vi "Main.vi"(8 "Error In":errorcluster, 9 "Pop-up New Error Dialogue Setting (Default = Pop-up Dialogue)":T1, 10 "The folder to store the Error Logs":path, 11 "Test Rig Name or Acronym":string) -> (0 "Error Out":errorcluster)   [LabVIEW 2023, in "Error Manager.lvlib"]
doc: "Error Manager. Asynchronous Module. User-facing GUI. Logs all errors to a log file.\n\nRecommended use: \n1. Start the Error Manager by calling this VI at application start prior to other asynchronous modules being started and prior to other start-up actions being performed (for example, prior to retrieving settings or limits from a file or from a database). This ensures that all parts of the app can report to the Error Manager any errors encountered during app start-up.\n\n2. Use Public API VIs to interact with this VI. For example, call 'Handle Error' to report an error to the asynchronous Error Manager module, or call 'Show Front Panel' to pop-up the Error Manager GUI to the user.\n\n3. Close the Error Manager by calling 'Close Module' during app shutdown, after all other shutdown operations have been completed (for example, after all other asynchronous modules have been stopped). This enables the Error Manager to log any errors that may happen during app shutdown.\n\nError in behaviour: This VI skips execution (does not execute) if 'error in' contains an error."
uses:
  Error Manager.lvlib
  Pop-up New Error Dialogue Setting (enum).ctl
  MHL Queue/Command (enum).ctl
  LogToFileQueue/Command (enum).ctl
  NewErrorDialogueLoopQueue/Command (enum).ctl
  New Error Dialogue GUI/New Error (To Be Displayed To User) (cluster).ctl
  Error Log/Error to be logged (cluster).ctl
  Error Log/Error Type (enum).ctl
  Reported Error (cluster).ctl
  Pop-up New Error Dialogue Instruction (enum).ctl
  Read-Unread Status (enum).ctl
  Error in current one-second interval (cluster).ctl
  <vilib>/Utility/error.llb/DialogType.ctl
  Error Log/ErrorLog.lvlib
  MHL Queue/MHL Queue.lvlib
  LogToFileQueue/LogToFileQueue.lvlib
  NewErrorDialogueLoopQueue/NewErrorDialogueLoopQueue.lvlib
  New Error Dialogue GUI/New Error Dialogue GUI.lvlib
panel:
  in  "Sizing Tool":bool
  in  "Mark error as read":bool
  in  "Mark all errors as read":bool
  in  "Display Order ComboBox":string(combo) caption="Display Order"
  out "Error Out":errorcluster
  in  "Open Error Logs Folder":bool
  in  "Open Error Log in Notepad":bool
  out "Error Log Filepath":string
  out "Full Error Message":string caption="Error Message Of Selected Error"
  in  "MCL":i32[](listbox) caption="Errors since app started"
  out "Close module?":bool
  out "EHL iteration":i32
  out "MHL iteration":i32
  out "Error Out":errorcluster
  # "The region below is invisible to the user. For developer use only."
  # "Input\nInputs to the VI"
  # "Development\ncontrols/indicators useful for development and testing, but which are not outputs of the VI"
  # "Output\nOutputs of the VI"
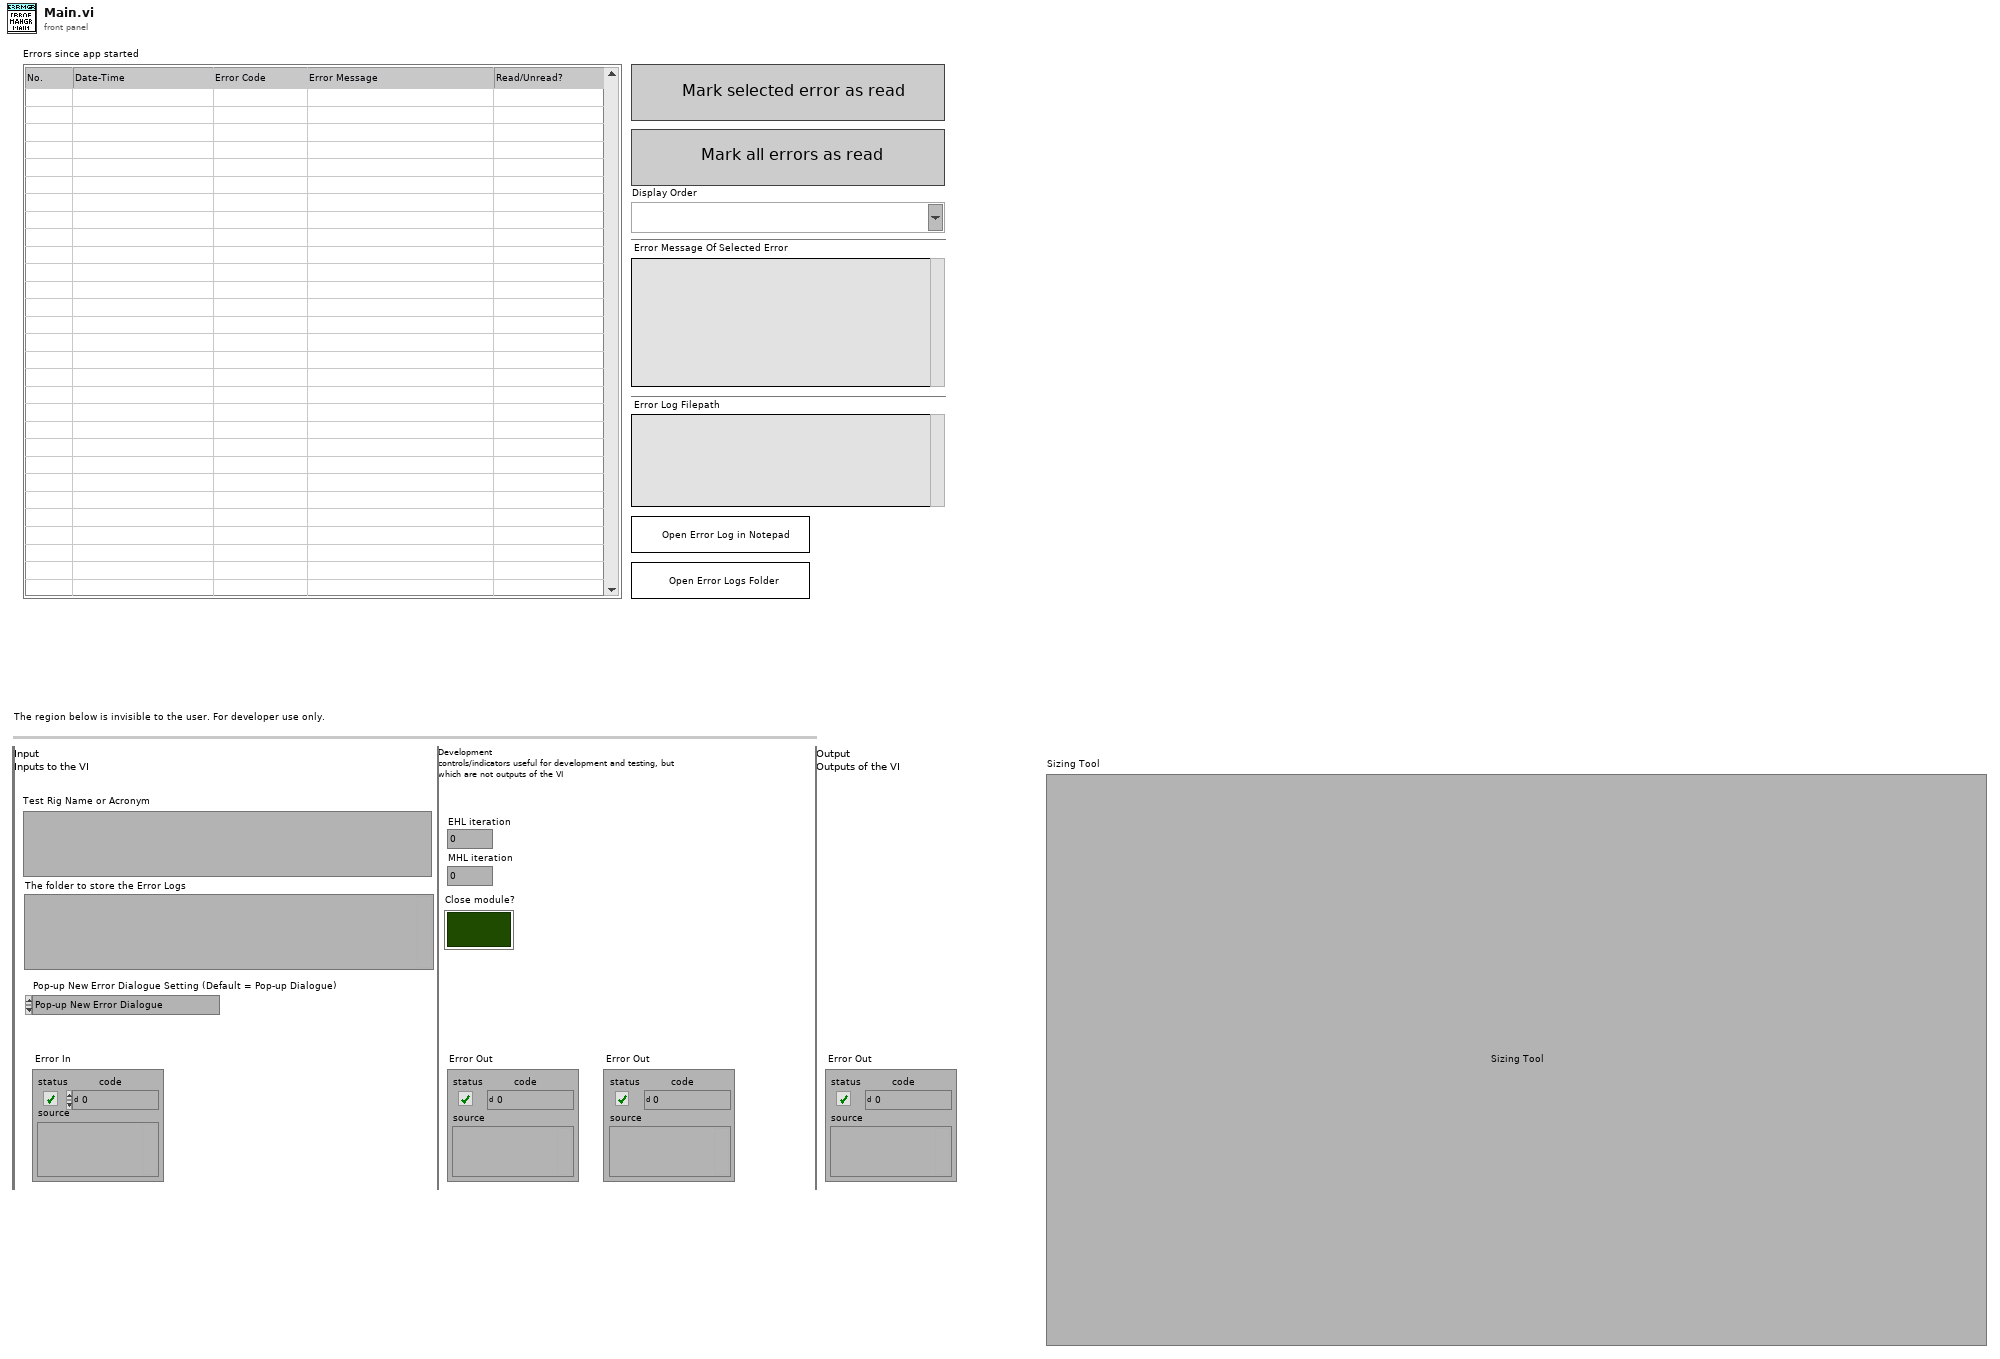
[diagram p1: front panel]
types:
  T1 = typedef "Error Manager.lvlib/Pop-up New Error Dialogue Setting (enum).ctl" = enum16{"Pop-up New Error Dialogue", "Don't pop-up New Error Dialogue"}
  T2 = typedef "Error Manager.lvlib/NewErrorDialogueLoopQueue.lvlib/Command (enum).ctl" = enum16{"Init Loop", "Close Loop", "Pop-up New Error Dialogue"}
  T3 = typedef "Error Manager.lvlib/LogToFileQueue.lvlib/Command (enum).ctl" = enum16{"Init Loop", "Close Loop", "Log Error"}
  T4 = typedef "Error Manager.lvlib/MHL Queue.lvlib/Command (enum).ctl" = enum16{"Init Module", "Close Module", "Internal Error", "Create Error Log File", "Show Front Panel", "Handle Error", "Refresh MCL", "MCL Value Change", "Mark Error As Read", "Mark All Errors As Read", "Change Display Order", "One-Second Interval Expired"}
  T5 = typedef "Error Manager.lvlib/ErrorLog.lvlib/Error to be logged (cluster).ctl" = cluster{"Error Type":T6, "Error Number":i32, "Timestamp":timestamp, "Error code":i32, "Error message":string}
  T6 = typedef "Error Manager.lvlib/ErrorLog.lvlib/Error Type (enum).ctl" = enum16{"New", "Identical to last logged error"}
  T7 = typedef "Error Manager.lvlib/Reported Error (cluster).ctl" = cluster{"Timestamp":timestamp, "Error code":i32, "Error message":string, "Pop-up New Error Dialogue Instruction":T8}
  T8 = typedef "Error Manager.lvlib/Pop-up New Error Dialogue Instruction (enum).ctl" = enum16{"Let Error Manager Decide (Default)", "Don't pop-up", "Pop-up"}
  T9 = typedef "Error Manager.lvlib/Read-Unread Status (enum).ctl" = enum16{"Unread", "Read"}
  T10 = typedef "Error Manager.lvlib/Module Data (cluster).ctl" = cluster{"Total no. of errors reported":i32, "Total no. of errors handled":i32, "Latest Handled Errors (chronological order)":T11[], "Display Order":T12, "Errors in current one-second interval":T13[], "ErrorMarkedAsRead":bool[]}
  T11 = typedef "Error Manager.lvlib/Handled Error (cluster).ctl" = cluster{"Error Number":i32, "Timestamp":timestamp, "Error code":i32, "Error message":string, "Read-Unread Status":T9}
  T12 = typedef "Error Manager.lvlib/Display Order (enum).ctl" = enum16{"Most Recent First (inverse-chronological)", "Oldest First (chronological)"}
  T13 = typedef "Error Manager.lvlib/Error in current one-second interval (cluster).ctl" = cluster{"Error code":i32, "No. of times error reported":u32, "No. of times error handled":u32}
  T14 = typedef "Error Manager.lvlib/New Error Dialogue GUI.lvlib/New Error (To Be Displayed To User) (cluster).ctl" = cluster{"Error Code":i32, "Error Message":string}
  T15 = typedef "DialogType.ctl" = u16
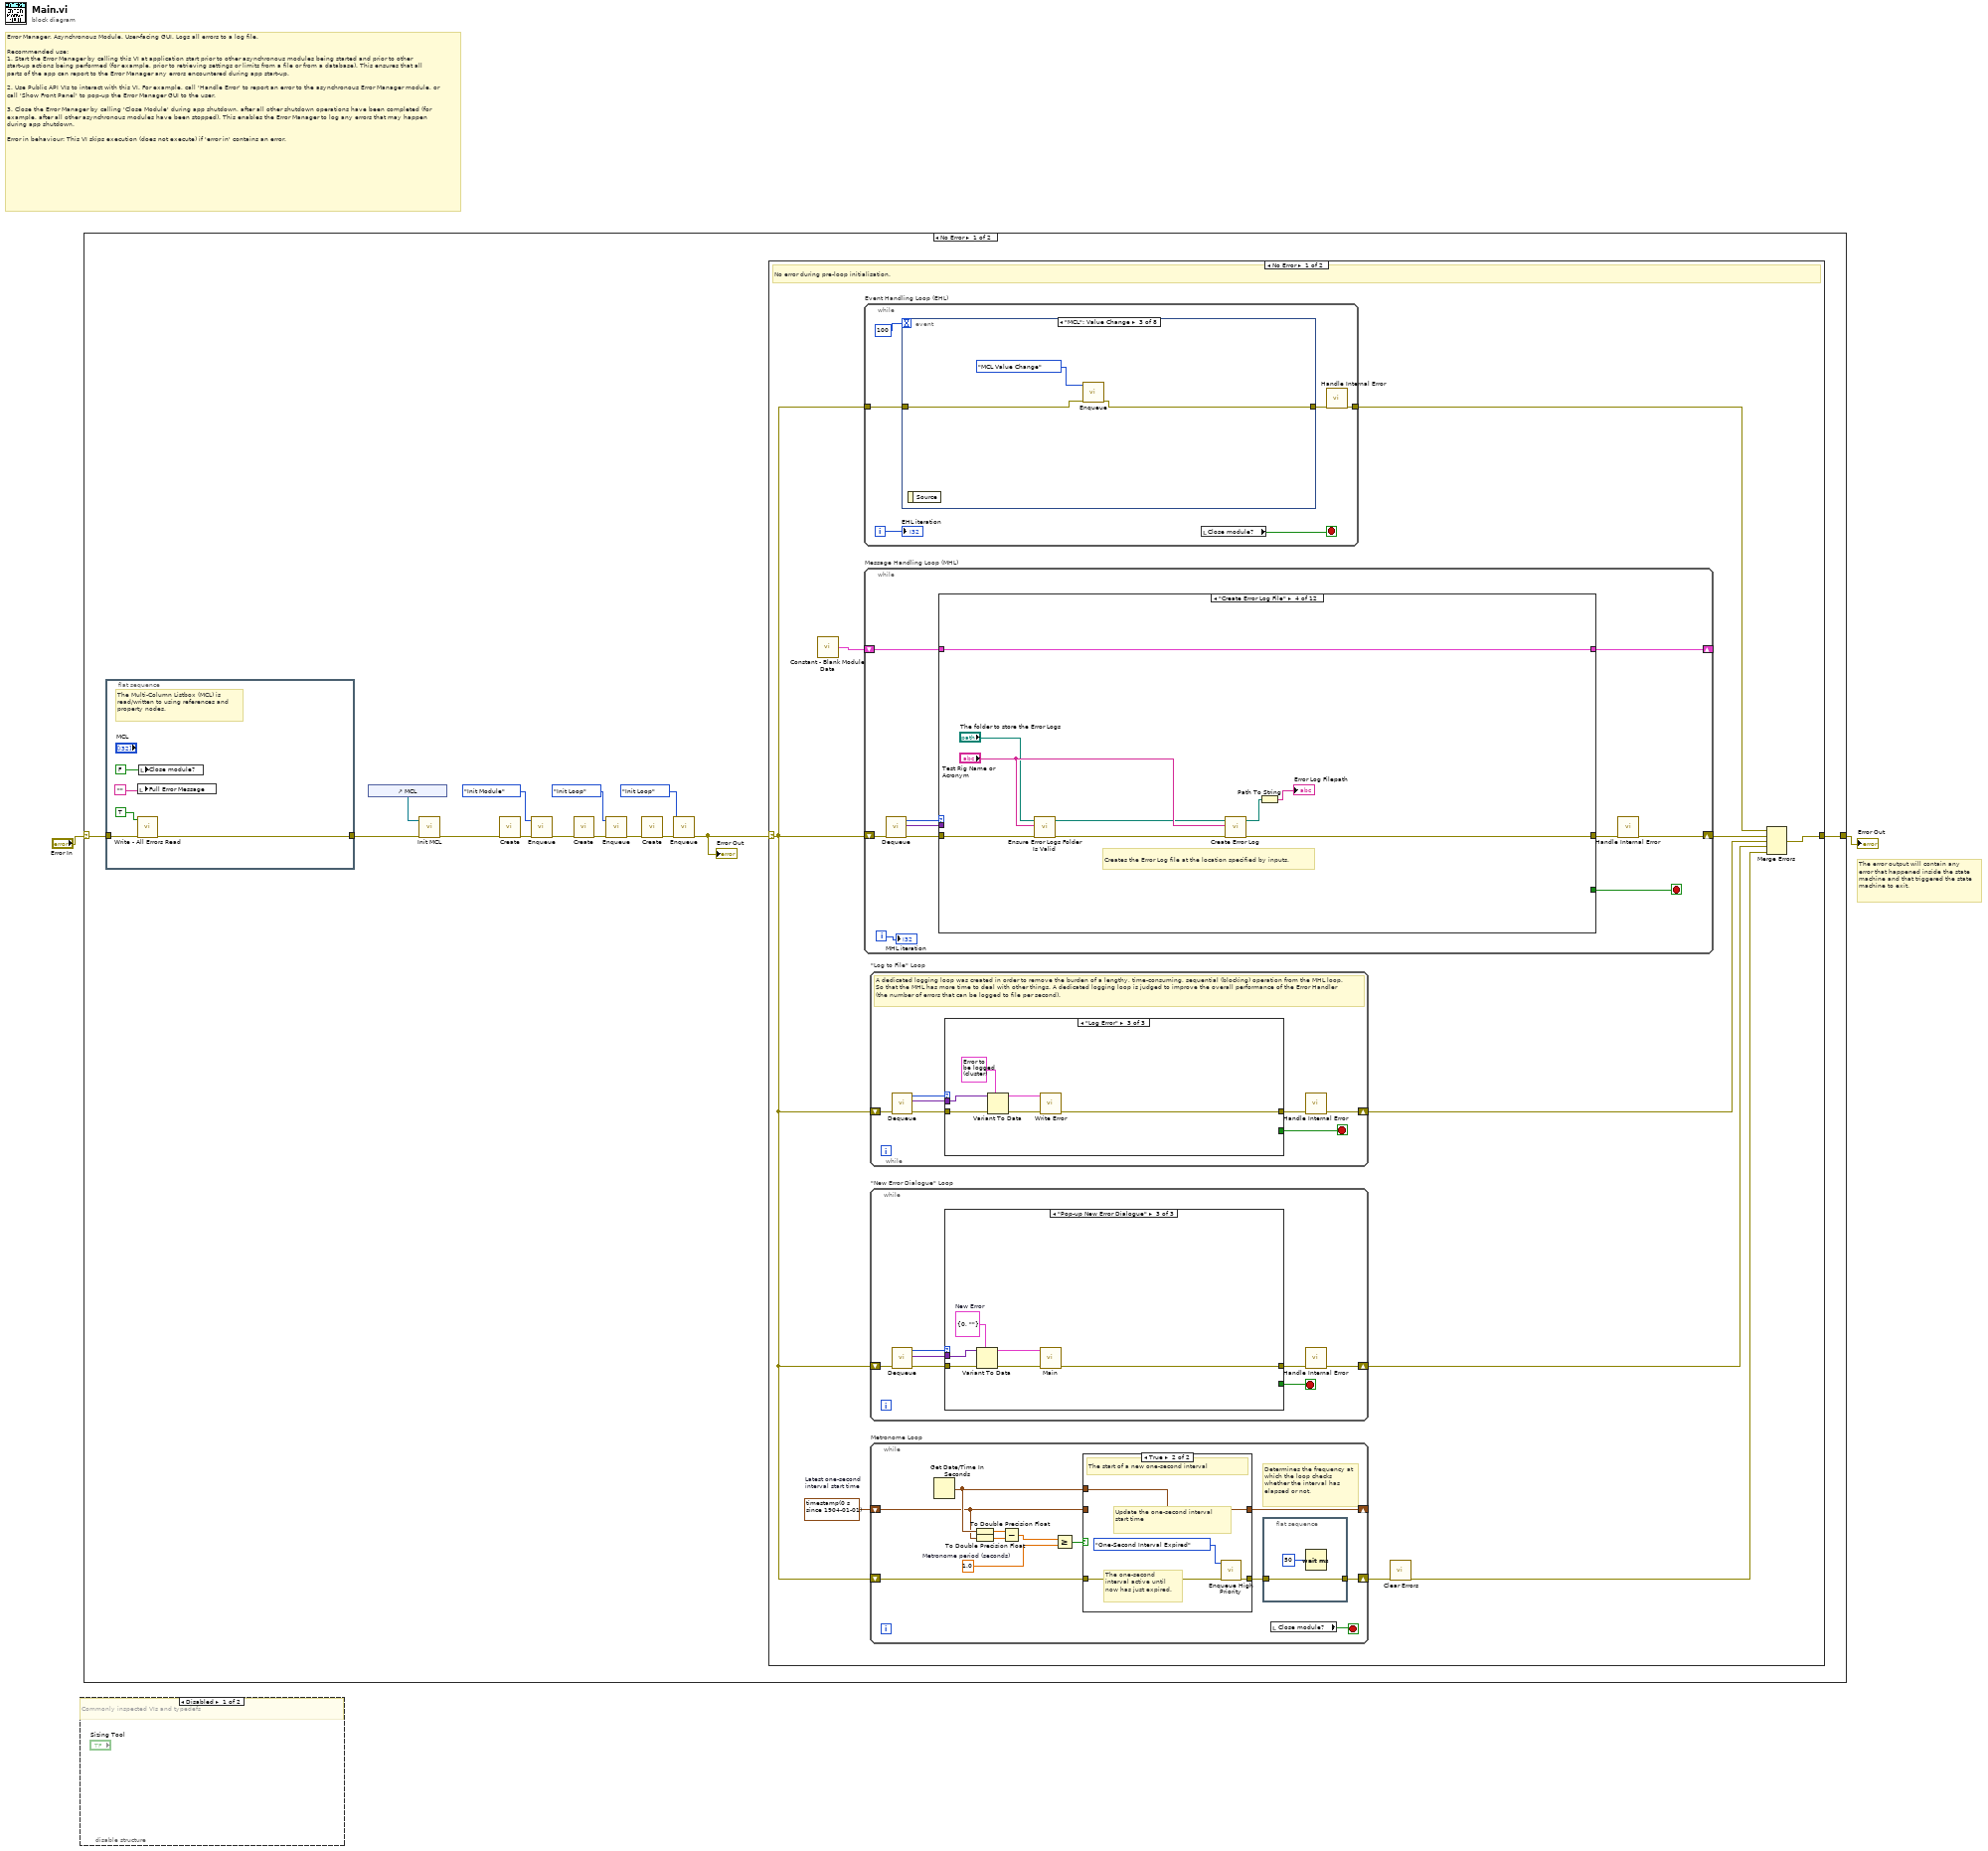
[diagram p0: block diagram]
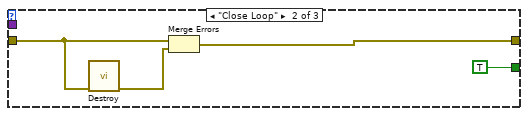
[diagram p3: hidden frame]
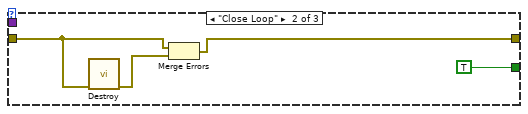
[diagram p5: hidden frame]
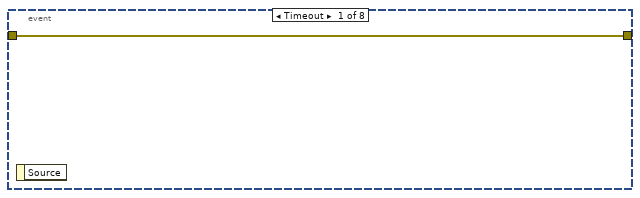
[diagram p6: hidden frame]
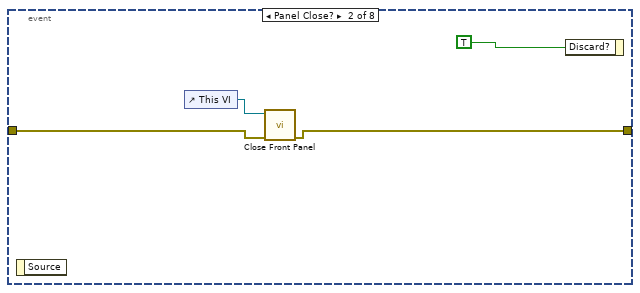
[diagram p7: hidden frame]
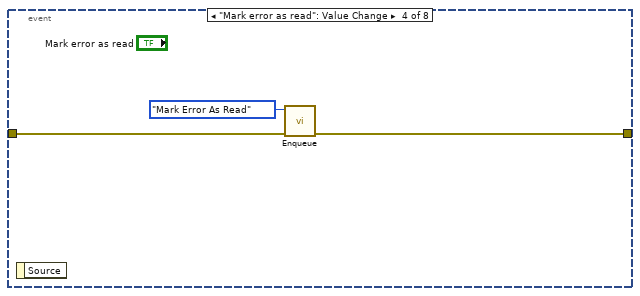
[diagram p8: hidden frame]
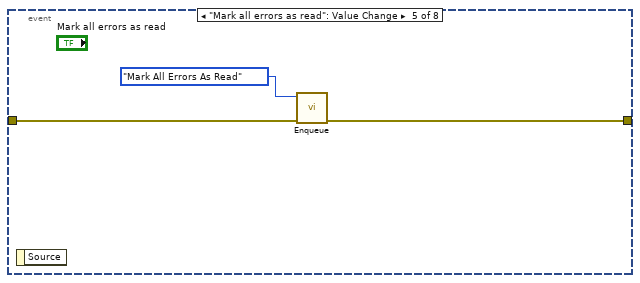
[diagram p9: hidden frame]
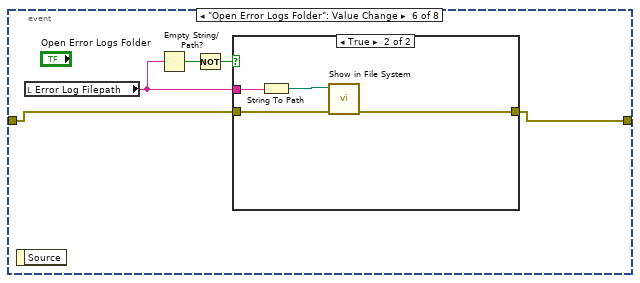
[diagram p10: hidden frame]
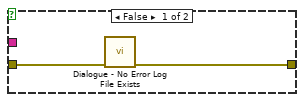
[diagram p11: hidden frame]
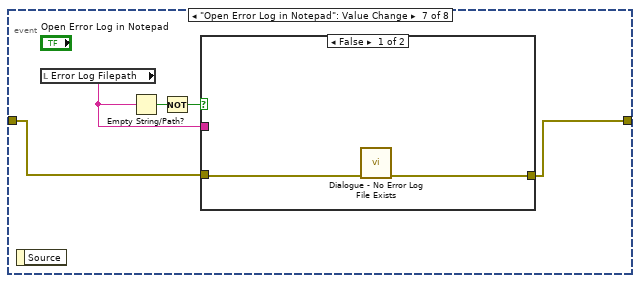
[diagram p12: hidden frame]
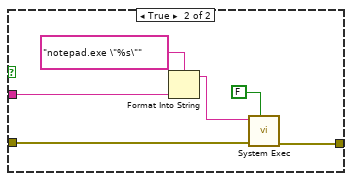
[diagram p13: hidden frame]
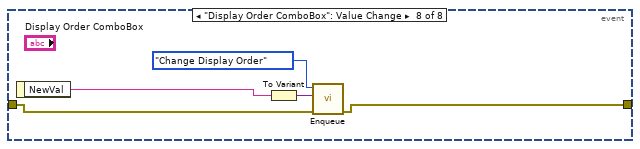
[diagram p14: hidden frame]
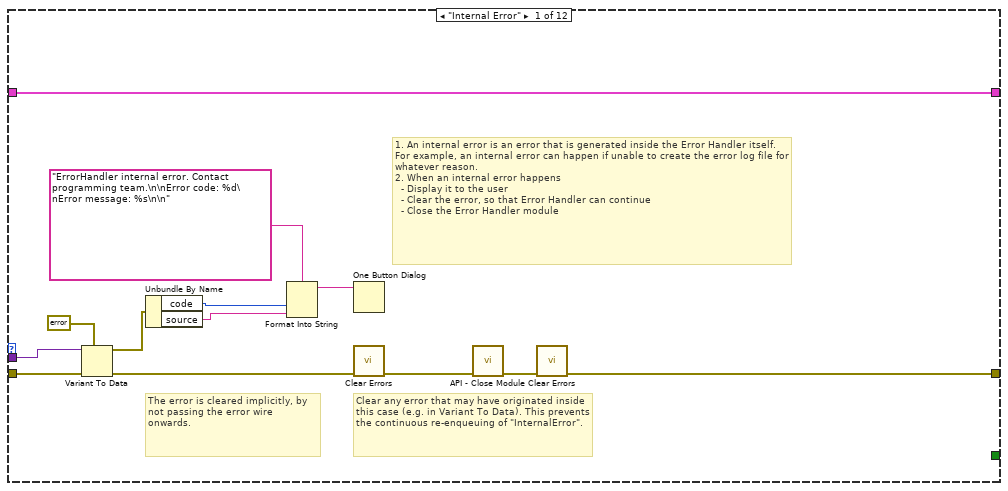
[diagram p15: hidden frame]
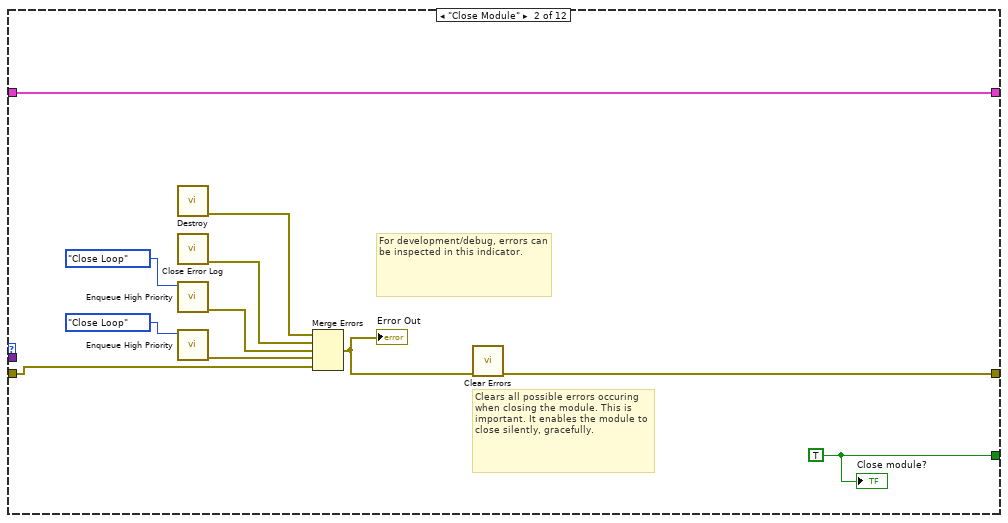
[diagram p16: hidden frame]
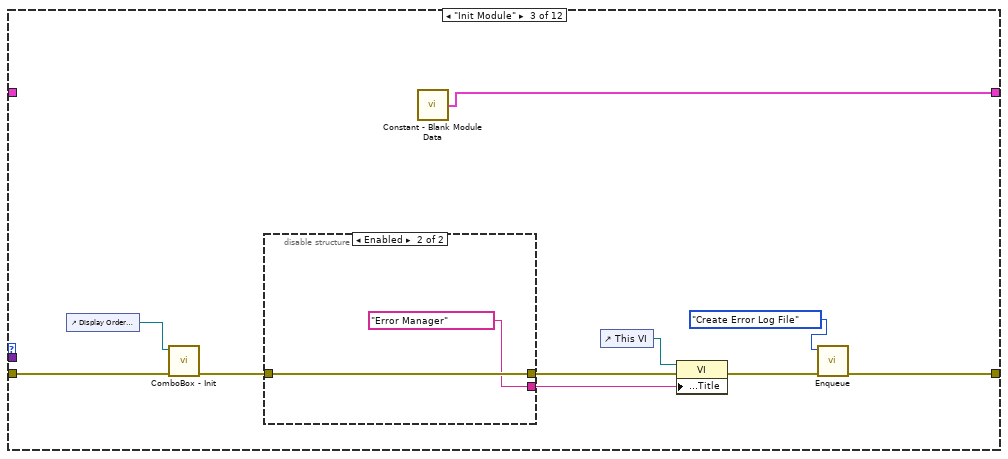
[diagram p17: hidden frame]
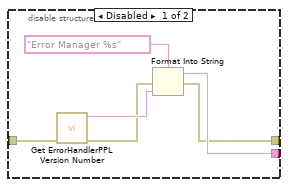
[diagram p18: hidden frame]
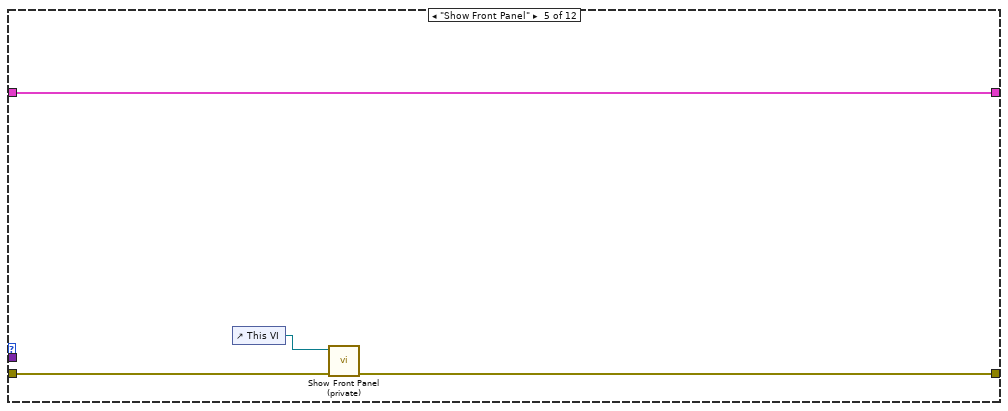
[diagram p19: hidden frame]
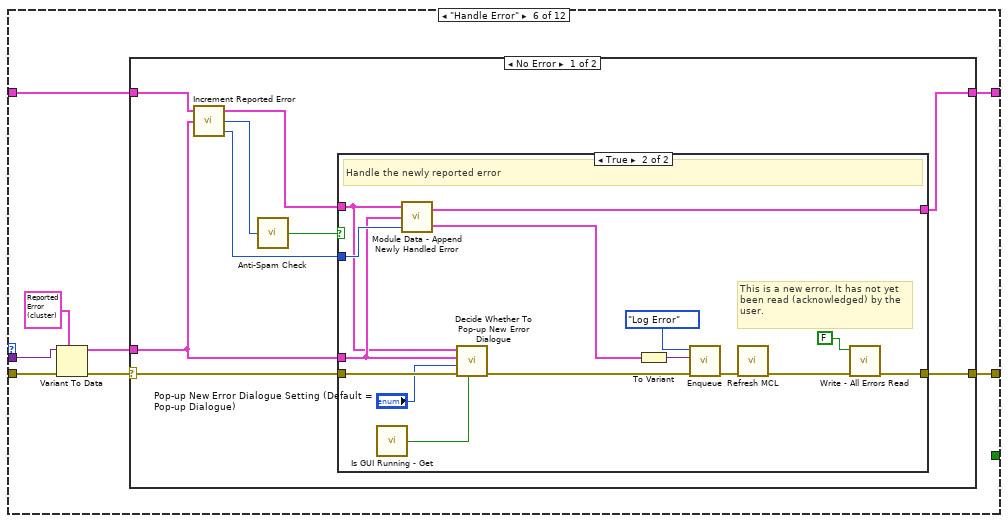
[diagram p20: hidden frame]
diagram:
  # "The error output will contain any error that happened inside the state machine and that triggered the state machine to exit."
  # "Error Manager. Asynchronous Module. User-facing GUI. Logs all errors to a log file.\n\nRecommended use: \n1. Start the Error Manager by calling this VI at application start prior to other asynchronous modules being started and prior to other start-up actions being performed (for example, prior to retrieving settings or limits from a file or from a database). This ensures that all parts of the app can report to the Error Manager any errors encountered during app start-up.\n\n2. Use Public API VIs to interact with this VI. For example, call 'Handle Error' to report an error to the asynchronous Error Manager module, or call 'Show Front Panel' to pop-up the Error Manager GUI to the user.\n\n3. Close the Error Manager by calling 'Close Module' during app shutdown, after all other shutdown operations have been completed (for example, after all other asynchronous modules have been stopped). This enables the Error Manager to log any errors that may happen during app shutdown.\n\nError in behaviour: This VI skips execution (does not execute) if 'error in' contains an error."
  n1 = disable-structure shown="Disabled" {
    frame Disabled {
      # "Commonly inspected VIs and typedefs"
    }
    frame Enabled {
    }
  }
  n2 = case shown="No Error" "Error In" {
    selector: "Error In" -> [w13 w377]
    tunnel: [w16 w377] -> w2
    frame No Error {
      n3 = flat-sequence {
        tunnel: [w20] -> w11
        tunnel: w13 -> [w19]
        frame #0 {
          # "The Multi-Column Listbox (MCL) is read/written to using references and property nodes."
          n4 = call "Write - All Errors Read.vi"("error in (no error)"=w19, "All Errors Read?"=TRUE) -> ("error out"=w20:errorcluster)  [unwired: 9 in]
          n5 = local write "Full Error Message"("") -> ()
          n6 = local write "Close module?"(FALSE ("Close module?")) -> ()
        }
      }
      n7 = control-ref of="MCL"() -> (w12:refnum<vi>)
      n8 = call "Init MCL.vi"("error in (no error)"=w11, "MCL Reference"=w12) -> ("error out"=w10:errorcluster)  [unwired: 9 in]
      n9 = call "Create.vi"("error in (no error)"=w10) -> ("error out"=w15:errorcluster)  [unwired: 10 in]
      n10 = call "Enqueue.vi"("error in (no error)"=w15, "Command"=Command_(enum)."Init Module") -> ("error out"=w14:errorcluster)  [unwired: 9 in]
      n11 = call "Create.vi"("error in (no error)"=w14) -> ("error out"=w8:errorcluster)  [unwired: 10 in]
      n12 = call "Enqueue.vi"("error in (no error)"=w8, "Command"=Command_(enum)."Init Loop") -> ("error out"=w7:errorcluster)  [unwired: 9 in]
      n13 = call "Create.vi"("error in (no error)"=w7) -> ("error out"=w5:errorcluster)  [unwired: 10 in]
      n14 = call "Enqueue.vi"("error in (no error)"=w5, "Command"=Command_(enum)."Init Loop") -> ("error out"=w4:errorcluster)  [unwired: 9 in]
      "Error Out" <- w4
      n15 = case shown="No Error" w4 {
        selector: w4 -> [w24 w376]
        tunnel: [w30 w375] -> w16
        frame No Error {
          w28 = timestamp(0 s since 1904-01-01)  # Latest one-second interval start time
          # "No error during pre-loop initialisation."
          n16 = call "Constant - Blank Module Data.vi"() -> ("Blank Module Data"=w26:T10)
          n17 = while "Event Handling Loop (EHL)" {
            tunnel: w24 -> [w70]
            tunnel: [w68] -> w29
            i -> [w73]
            stop <- w71 stop-if-true
            n18 = event shown="[2] \"MCL\": Value Change" {
              selector: _ -> [_ _ _ _ _ _ _ _]
              dyn-events: _ -> [_ _ _ _ _ _ _ _]
              timeout: 100 -> [_ _ _ _ _ _ _ _]
              tunnel: w70 -> [w74 w76 w81 w84 w87 w89 w100 w116]
              tunnel: [w74 w75 w80 w83 w86 w88 w99 w115] -> w69
              event Timeout {
                n19 = event-data() -> ()  [unwired: 1 in, 1 out]
              }
              event Panel Close? {
                n20 = event-data() -> ()  [unwired: 1 in, 1 out]
                n21 = control-ref of="This VI"() -> (w77:refnum<vi>)
                n22 = call "Close Front Panel.vi"("Error In"=w76, "VI Reference"=w77) -> ("Error Out"=w75:errorcluster)  [unwired: 9 in]
                n23 = event-data("Discard?"=TRUE) -> ()  [unwired: 1 in, 1 out]
              }
              event "MCL": Value Change {
                n24 = event-data() -> ()  [unwired: 1 in, 1 out]
                n25 = call "Enqueue.vi"("error in (no error)"=w81, "Command"=Command_(enum)."MCL Value Change") -> ("error out"=w80:errorcluster)  [unwired: 9 in]
              }
              event "Mark error as read": Value Change {
                n26 = event-data() -> ()  [unwired: 1 in, 1 out]
                n27 = call "Enqueue.vi"("error in (no error)"=w84, "Command"=Command_(enum)."Mark Error As Read") -> ("error out"=w83:errorcluster)  [unwired: 9 in]
              }
              event "Mark all errors as read": Value Change {
                n28 = event-data() -> ()  [unwired: 1 in, 1 out]
                n29 = call "Enqueue.vi"("error in (no error)"=w87, "Command"=Command_(enum)."Mark All Errors As Read") -> ("error out"=w86:errorcluster)  [unwired: 9 in]
              }
              event "Open Error Logs Folder": Value Change {
                n30 = event-data() -> ()  [unwired: 1 in, 1 out]
                n31 = local read "Error Log Filepath"() -> (w90:string)
                n32 = Empty String/Path?(string/path=w90) -> (empty?=w92:bool)
                n33 = Not(x=w92) -> (.not. x?=w91:bool)
                n34 = case shown="True" w91 {
                  tunnel: w90 -> [_ w97]
                  tunnel: w89 -> [w93 w96]
                  tunnel: [w94 w95] -> w88
                  frame False {
                    n35 = call "Dialogue - No Error Log File Exists.vi"("error in (no error)"=w93) -> ("error out"=w94:errorcluster)  [unwired: 10 in]
                  }
                  frame True {
                    n36 = String To Path(string=w97) -> (path=w98:path)
                    n37 = call <vilib>:"Show in File System.vi"("error in (no error)"=w96, "file or directory path"=w98) -> ("error out"=w95:errorcluster)  [unwired: 9 in]
                  }
                }
              }
              event "Open Error Log in Notepad": Value Change {
                n38 = event-data() -> ()  [unwired: 1 in, 1 out]
                n39 = local read "Error Log Filepath"() -> (w101:string)
                n40 = Empty String/Path?(string/path=w101) -> (empty?=w102:bool)
                n41 = Not(x=w102) -> (.not. x?=w103:bool)
                n42 = case shown="False" w103 {
                  tunnel: w100 -> [w105 w109]
                  tunnel: [w104 w108] -> w99
                  tunnel: w101 -> [_ w107]
                  frame False {
                    n43 = call "Dialogue - No Error Log File Exists.vi"("error in (no error)"=w105) -> ("error out"=w104:errorcluster)  [unwired: 10 in]
                  }
                  frame True {
                    n44 = Format Into String(format string="notepad.exe \"%s\"", w107) -> (resulting string=w110:string)  [unwired: 2 in, 1 out]
                    n45 = call <vilib>:"System Exec.vi"("wait until completion? (T)"=FALSE, "error in (no error)"=w109, "command line"=w110) -> ("error out"=w108:errorcluster)  [unwired: 5 in, 3 out]
                  }
                }
              }
              event "Display Order ComboBox": Value Change {
                n46 = event-data() -> ("NewVal"=w114:string)  [unwired: 1 in]
                n47 = To Variant(anything=w114) -> (Variant=w113:variant)
                n48 = call "Enqueue.vi"("error in (no error)"=w116, "Data"=w113, "Command"=Command_(enum)."Change Display Order") -> ("error out"=w115:errorcluster)  [unwired: 8 in]
              }
            }
            n49 = local read "Close module?"() -> (w71:bool)
            n50 = call "Handle Internal Error.vi"("error in (no error)"=w69) -> ("error out"=w68:errorcluster)  [unwired: 10 in]
            "EHL iteration" <- w73
          }
          n51 = while "Message Handling Loop (MHL)" {
            shift-right: [w120] -> w31
            shift-left: w24 -> [w124]
            shift-right: [w122] -> _
            shift-left: w26 -> [w117]
            i -> [w123]
            stop <- w126 stop-if-true
            n52 = call "Dequeue.vi"("error in (no error)"=w124) -> ("error out"=w125:errorcluster, "Data"=w118:variant, "Command"=w119:T4)  [unwired: 8 in]
            n53 = case shown="\"Create Error Log File\"" w119 {
              tunnel: w125 -> [w136 w142 w159 w174 w179 w189 w223 w235 w251 w287 w340 w353]
              tunnel: [w127 w146 w160 w173 w180 w186 w222 w235 w239 w276 w335 w352] -> w121
              tunnel: [_ w148 _ _ _ _ _ _ _ _ _ _] -> w126
              tunnel: w118 -> [w134 _ _ _ _ w187 _ _ _ _ w331 _]
              tunnel: w117 -> [w132 w149 _ w177 w181 w183 w226 w234 w246 w282 w333 w349]
              tunnel: [w132 w149 w155 w177 w181 w184 w226 w234 w244 w281 w334 w350] -> w122
              frame "Internal Error" {
                # "The error is cleared implicitly, by not passing the error wire onwards."
                # "1. An internal error is an error that is generated inside the Error Handler itself. For example, an internal error can happen if unable to create the error log file for whatever reason.\n2. When an internal error happens\n  - Display it to the user\n  - Clear the error, so that Error Handler can continue\n  - Close the Error Handler module"
                # "Clear any error that may have originated inside this case (e.g. in Variant To Data). This prevents the continuous re-enqueuing of \"InternalError\"."
                n54 = Variant To Data(error in=w136, type=errorcluster {"status"=FALSE, "code"=0, "source"=""} ("error constant"), Variant=w134) -> (data=w131:errorcluster, error out=w133:errorcluster)
                n55 = Unbundle By Name(w131) -> ("code"=w137:i32, "source"=w130:string)
                n56 = Format Into String(format string="ErrorHandler internal error. Contact programming team.\n\nError code: %d\nError message: %s\n\n" ("Warning"), w137, w130) -> (resulting string=w138:string)  [unwired: 2 in, 1 out]
                n57 = One Button Dialog(message=w138) -> ()  [unwired: 1 in, 1 out]
                n58 = call <vilib>:"Clear Errors.vi"("error in (no error)"=w133) -> ("error out"=w129:errorcluster)  [unwired: 5 in, 1 out]
                n59 = call "API - Close Module.vi"("error in"=w129) -> ("error out"=w128:errorcluster)  [unwired: 10 in]
                n60 = call <vilib>:"Clear Errors.vi"("error in (no error)"=w128) -> ("error out"=w127:errorcluster)  [unwired: 5 in, 1 out]
              }
              frame "Close Module" {
                w148 = TRUE
                # "For development/debug, errors can be inspected in this indicator."
                # "Clears all possible errors occuring when closing the module. This is important. It enables the module to close silently, gracefully."
                n61 = call "Destroy.vi"() -> ("error out"=w150:errorcluster)  [unwired: 9 in, 2 out]
                n62 = call "Close Error Log.vi"() -> ("error out"=w147:errorcluster)  [unwired: 11 in]
                n63 = call "Enqueue High Priority.vi"("Command"=Command_(enum)."Close Loop") -> ("error out"=w143:errorcluster)  [unwired: 10 in]
                n64 = call "Enqueue High Priority.vi"("Command"=Command_(enum)."Close Loop") -> ("error out"=w141:errorcluster)  [unwired: 10 in]
                n65 = Merge Errors(w150, w147, w143, w141, w142) -> (w145:errorcluster)
                "Error Out" <- w145
                n66 = call <vilib>:"Clear Errors.vi"("error in (no error)"=w145) -> ("error out"=w146:errorcluster)  [unwired: 5 in, 1 out]
                "Close module?" <- w148
              }
              frame "Init Module" {
                n67 = control-ref of="Display Order ComboBox"() -> (w157:refnum<vi>)
                n68 = call "ComboBox - Init.vi"("error in (no error)"=w159, "ComboBox Ref"=w157) -> ("error out"=w158:errorcluster)  [unwired: 9 in]
                n69 = disable-structure shown="Enabled" {
                  disable-tunnel: w158 -> [w166 w168]
                  disable-tunnel: [w163 "Error Manager"] -> w152
                  disable-tunnel: [w161 w168] -> w151
                  frame Disabled {
                    n70 = call "Get ErrorHandlerPPL Version Number.vi"("error in"=w166) -> ("error out"=w162:errorcluster, "ErrorHandlerPPL Version Number"=w164:string)  [unwired: 9 in]
                    n71 = Format Into String(format string="Error Manager %s", error in=w162, w164) -> (resulting string=w163:string, error out=w161:errorcluster)  [unwired: 1 in]
                  }
                  frame Enabled {
                  }
                }
                n72 = call "Constant - Blank Module Data.vi"() -> ("Blank Module Data"=w155:T10)
                n73 = control-ref of="This VI"() -> (w153:refnum<vi>)
                n74 = property class="VI"(reference=w153, error in=w151, "Front Panel.Title"=w152) -> (error out=w154:errorcluster)  [unwired: 1 out]
                n75 = call "Enqueue.vi"("error in (no error)"=w154, "Command"=Command_(enum)."Create Error Log File") -> ("error out"=w160:errorcluster)  [unwired: 9 in]
              }
              frame "Create Error Log File" {
                # "Creates the Error Log file at the location specified by inputs."
                n76 = call "Ensure Error Logs Folder Is Valid.vi"("Error In"=w174, "Test Rig Name or Acronym"="Test Rig Name or Acronym", "Error Logs Folder (as provided by calling application)"="The folder to store the Error Logs") -> ("Error Out"=w172:errorcluster, "Error Logs Folder (valid)"=w169:path)  [unwired: 7 in]
                n77 = call "Create Error Log.vi"("error in (no error)"=w172, "Jig name (or acronym)"="Test Rig Name or Acronym", "The folder to store the Error Logs"=w169) -> ("error out"=w173:errorcluster, "Full file path of the Error Log"=w176:path)  [unwired: 6 in, 1 out]
                n78 = Path To String(path=w176) -> (string=→"Error Log Filepath":string)
              }
              frame "Show Front Panel" {
                n79 = control-ref of="This VI"() -> (w178:refnum<vi>)
                n80 = call "Show Front Panel (private).vi"("Error In"=w179, "VI Reference"=w178) -> ("Error Out"=w180:errorcluster)  [unwired: 9 in]
              }
              frame "Handle Error" {
                n81 = Variant To Data(error in=w189, type=T7 {"Timestamp"=timestamp(0 s since 1904-01-01), "Error code"=0, "Error message"="", "Pop-up New Error Dialogue Instruction"=enum."Let Error Manager Decide (Default)"} ("Error"), Variant=w187) -> (data=w185:T7, error out=w188:errorcluster)
                n82 = case shown="No Error" w188 {
                  selector: w188 -> [w197 w219]
                  tunnel: [w196 w217] -> w186
                  tunnel: w185 -> [w193 _]
                  tunnel: [w198 w216] -> w184
                  tunnel: w183 -> [w194 w216]
                  frame No Error {
                    n83 = call "Increment Reported Error.vi"("Newly Reported Error"=w193, "Module Data in"=w194) -> ("Index of the newly reported error in the OSI data structure"=w190:i32, "No. of times the error was handled in the last second"=w192:u32, "Module Data out (OSI data updated)"=w195:T10)  [unwired: 1 in]
                    n84 = call "Anti-Spam Check.vi"("No. of times the error has been handled in current One-Second Interval"=w192) -> ("Need to handle this error?"=w191:bool)
                    n85 = case shown="True" w191 {
                      tunnel: [w200 w205] -> w198
                      tunnel: w197 -> [w199 w206]
                      tunnel: [w199 w213] -> w196
                      tunnel: w195 -> [w200 w201]
                      tunnel: w193 -> [_ w204]
                      tunnel: w190 -> [_ w211]
                      frame False {
                        # "Do nothing."
                        # "The newly reported error is spam. Don't handle it."
                      }
                      frame True {
                        # "This is a new error. It has not yet been read (acknowledged) by the user."
                        # "Handle the newly reported error"
                        n86 = call "Is GUI Running - Get.vi"() -> ("Is GUI Running?"=w202:bool)
                        n87 = call "Module Data - Append Newly Handled Error.vi"("Index of the newly reported error in the OSI data structure"=w211, "Newly Reported Error"=w204, "Module Data in"=w201) -> ("Error to be logged"=w209:T5, "Module Data out (Error appended)"=w205:T10)
                        n88 = call "Decide Whether To Pop-up New Error Dialogue.vi"("Is New Error Dialogue GUI Running Already?"=w202, "Error In"=w206, "Pop-up New Error Dialogue Setting (Default = Pop-up Dialogue)"="Pop-up New Error Dialogue Setting (Default = Pop-up Dialogue)", "Newly Reported Error"=w204, "Module Data in"=w201) -> ("Error Out"=w207:errorcluster)  [unwired: 6 in]
                        n89 = To Variant(anything=w209) -> (Variant=w208:variant)
                        n90 = call "Enqueue.vi"("error in (no error)"=w207, "Data"=w208, "Command"=Command_(enum)."Log Error") -> ("error out"=w215:errorcluster)  [unwired: 8 in]
                        n91 = call "Refresh MCL.vi"("error in (no error)"=w215) -> ("error out"=w214:errorcluster)  [unwired: 10 in]
                        n92 = call "Write - All Errors Read.vi"("error in (no error)"=w214, "All Errors Read?"=FALSE) -> ("error out"=w213:errorcluster)  [unwired: 9 in]
                      }
                    }
                  }
                  frame Error {
                    # "This case should never execute. If it executes, fix the issue by making sure that this case is accessed only by calling the \"HandleError.vi\" API VI."
                    n93 = call <vilib>:"Clear Errors.vi"("error in (no error)"=w219) -> ("error out"=w218:errorcluster)  [unwired: 5 in, 1 out]
                    n94 = call "Throw Error (no overwrite).vi"("error in"=w218, "Error Message (\"\")"="Assertion. Unable to convert variant to \"Error\" typedef cluster. There is a bug in the code. Contact programming team.") -> ("error out"=w217:errorcluster)  [unwired: 9 in]
                  }
                }
              }
              frame "Refresh MCL" {
                # "#todo\nIs Error MarkedAsRead needed?"
                n95 = Unbundle By Name(w226) -> ("Latest Handled Errors (chronological order)"=w224:T11[], "Display Order"=w221:T12)  [unwired: 1 out]
                n96 = control-ref of="MCL"() -> (w225:refnum<vi>)
                n97 = call "Refresh MCL (action).vi"("error in (no error)"=w223, "Display Order"=w221, "Errors To Display"=w224, "MCL Reference"=w225) -> ("error out"=w222:errorcluster)  [unwired: 7 in]
              }
              frame "MCL Value Change" {
                n98 = Unbundle By Name(w234) -> ("Latest Handled Errors (chronological order)"=w228:T11[], "Display Order"=w229:T12)
                n99 = local read "MCL"() -> (w231:i32[])
                n100 = Index Array(array=w231) -> (element=w230:i32)  [unwired: 1 in]
                n101 = case shown="\"Most Recent First (inverse-chronological)\", Default" w229 {
                  tunnel: w228 -> [w237 w238]
                  tunnel: [w236 w238] -> w227
                  frame "Most Recent First (inverse-chronological)", Default {
                    n102 = Reverse 1D Array(array=w237) -> (reversed array=w236:T11[])
                  }
                  frame "Oldest First (chronological)" {
                  }
                }
                n103 = Index Array(array=w227, index=w230) -> (element=w233:T11)
                n104 = Unbundle By Name(w233) -> ("Error message"=→"Full Error Message":string)
              }
              frame "Mark Error As Read" {
                n105 = control-ref of="MCL"() -> (w249:refnum<vi>)
                n106 = Unbundle By Name(w246) -> ("Latest Handled Errors (chronological order)"=w248:T11[], "Display Order"=w243:T12, "ErrorMarkedAsRead"=w242:bool[])
                n107 = call "MCL - Get Selected Rows.vi"("error in (no error)"=w251, "MCL Reference"=w249) -> ("error out"=w250:errorcluster, "Index of first selected row"=w247:i32)  [unwired: 5 in, 3 out]
                n108 = call "MCL - Set Row Background Colour - Read.vi"("error in (no error)"=w250, "Row index"=w247, "MCL"=w249) -> ("error out"=w240:errorcluster)  [unwired: 8 in]
                n109 = case shown="\"Oldest First (chronological)\"" w243 {
                  tunnel: w248 -> [w264 w270]
                  tunnel: w247 -> [w255 w267]
                  tunnel: [w259 w269] -> w245
                  tunnel: w242 -> [w257 w268]
                  tunnel: [w252 w266] -> w241
                  frame "Most Recent First (inverse-chronological)", Default {
                    # "Reverse array, update status then return array to original before bundling"
                    n110 = Reverse 1D Array(array=w264) -> (reversed array=w261:T11[])
                    n111 = Reverse 1D Array(array=w257) -> (reversed array=w256:bool[])
                    n112 = Index Array(array=w261, index=w255) -> (element=w263:T11)
                    n113 = Replace Array Subset(array=w256, new element=TRUE ("new element/subarray"), index=w255) -> (w253:bool[])
                    n114 = Bundle By Name(cluster=w263, "Read-Unread Status"=Read-Unread_Status_(enum)."Read") -> (w260:T11)
                    n115 = Reverse 1D Array(array=w253) -> (reversed array=w252:bool[])
                    n116 = Replace Array Subset(array=w261, new element=w260, index=w255) -> (w258:T11[])
                    n117 = Reverse 1D Array(array=w258) -> (reversed array=w259:T11[])
                  }
                  frame "Oldest First (chronological)" {
                    # "Update status in current orientation"
                    n118 = Index Array(array=w270, index=w267) -> (element=w273:T11)
                    n119 = Bundle By Name(cluster=w273, "Read-Unread Status"=Read-Unread_Status_(enum)."Read") -> (w271:T11)
                    n120 = Replace Array Subset(array=w270, new element=w271, index=w267) -> (w269:T11[])
                    n121 = Replace Array Subset(array=w268, new element=TRUE ("new element/subarray"), index=w267) -> (w266:bool[])
                  }
                }
                n122 = Bundle By Name(cluster=w246, "Latest Handled Errors (chronological order)"=w245, "ErrorMarkedAsRead"=w241) -> (w244:T10)
                n123 = call "Refresh MCL.vi"("error in (no error)"=w240) -> ("error out"=w239:errorcluster)  [unwired: 10 in]
              }
              frame "Mark All Errors As Read" {
                n124 = control-ref of="MCL"() -> (w284:refnum<vi>)
                n125 = Unbundle By Name(w282) -> ("Latest Handled Errors (chronological order)"=w283:T11[], "Display Order"=w278:T12, "ErrorMarkedAsRead"=w274:bool[])
                n126 = call "Write - All Errors Read.vi"("error in (no error)"=w287, "All Errors Read?"=TRUE) -> ("error out"=w285:errorcluster)  [unwired: 9 in]
                n127 = call "Get Row Indexes Of Unread Errors.vi"("Is Error Read?"=w274) -> ("Row Index Of Unread Errors"=w275:i32[])
                n128 = case shown="\"Most Recent First (inverse-chronological)\"" w278 {
                  tunnel: w285 -> [w295 w315]
                  tunnel: [w294 w314] -> w277
                  tunnel: w284 -> [w293 w313]
                  tunnel: w275 -> [w292 w310]
                  tunnel: w283 -> [w291 w312]
                  tunnel: [w290 w309] -> w280
                  tunnel: w274 -> [w289 w311]
                  tunnel: [w288 w308] -> w279
                  frame "Oldest First (chronological)" {
                    n129 = for {
                      shift-right: [w306] -> w294
                      shift-left: w295 -> [w307]
                      tunnel: w293 -> [w305]
                      tunnel: w292 -> [w298] mode=indexing
                      shift-right: [w300] -> w290
                      shift-left: w291 -> [w302]
                      shift-right: [w296] -> w288
                      shift-left: w289 -> [w299]
                      n130 = Index Array(array=w302, index=w298) -> (element=w301:T11)
                      n131 = Bundle By Name(cluster=w301, "Read-Unread Status"=Read-Unread_Status_(enum)."Read") -> (w303:T11)
                      n132 = call "MCL - Set Row Background Colour - Read.vi"("error in (no error)"=w307, "Row index"=w298, "MCL"=w305) -> ("error out"=w306:errorcluster)  [unwired: 8 in]
                      n133 = Replace Array Subset(array=w302, new element=w303, index=w298) -> (w300:T11[])
                      n134 = Replace Array Subset(array=w299, new element=TRUE ("new element/subarray"), index=w298) -> (w296:bool[])
                    }
                  }
                  frame "Most Recent First (inverse-chronological)" {
                    n135 = for {
                      shift-right: [w329] -> w314
                      shift-left: w315 -> [w330]
                      tunnel: w313 -> [w328]
                      tunnel: w310 -> [w318] mode=indexing
                      shift-right: [w323] -> w309
                      shift-left: w312 -> [w325]
                      shift-right: [w321] -> w308
                      shift-left: w311 -> [w320]
                      n136 = Index Array(array=w325, index=w318) -> (element=w324:T11)
                      n137 = Array Size(array=w320) -> (size(s)=w319:i32)
                      n138 = Bundle By Name(cluster=w324, "Read-Unread Status"=Read-Unread_Status_(enum)."Read") -> (w326:T11)
                      n139 = Subtract(x=w319, y=w318) -> (x-y=w317:i32)
                      n140 = Decrement(x=w317) -> (x-1=w316:i32)
                      n141 = call "MCL - Set Row Background Colour - Read.vi"("error in (no error)"=w330, "Row index"=w316, "MCL"=w328) -> ("error out"=w329:errorcluster)  [unwired: 8 in]
                      n142 = Replace Array Subset(array=w325, new element=w326, index=w318) -> (w323:T11[])
                      n143 = Replace Array Subset(array=w320, new element=TRUE ("new element/subarray"), index=w318) -> (w321:bool[])
                    }
                  }
                }
                n144 = Bundle By Name(cluster=w282, "Latest Handled Errors (chronological order)"=w280, "ErrorMarkedAsRead"=w279) -> (w281:T10)
                n145 = call "Refresh MCL.vi"("error in (no error)"=w277) -> ("error out"=w276:errorcluster)  [unwired: 10 in]
              }
              frame "Change Display Order" {
                # "Raises error if unable to convert string to enum."
                n146 = Variant To Data(error in=w340, type="", Variant=w331) -> (data=w336:string, error out=w339:errorcluster)
                n147 = call "ComboBox - Convert String To Enum.vi"("error in (no error)"=w339, "Display Order (ComboBox string)"=w336) -> ("error out"=w337:errorcluster, "Display Order (enum)"=w332:T12)  [unwired: 8 in]
                n148 = case shown="No Error" w337 {
                  selector: w337 -> [w345 w347]
                  tunnel: [w344 w347] -> w335
                  tunnel: w333 -> [w343 w346]
                  tunnel: [w342 w346] -> w334
                  tunnel: w332 -> [w341 _]
                  frame No Error {
                    n149 = Bundle By Name(cluster=w343, "Display Order"=w341) -> (w342:T10)
                    n150 = call "Refresh MCL.vi"("error in (no error)"=w345) -> ("error out"=w344:errorcluster)  [unwired: 10 in]
                  }
                  frame Error {
                  }
                }
              }
              frame "One-Second Interval Expired" {
                w348 = T13[] []  # Blank
                # "Refresh (clear) the errors accumulated in the last one-second interval."
                # "This case plays a role in the implementation of 'anti-spam' functionality."
                n151 = Unbundle By Name(w349) -> ("Errors in current one-second interval"=w351:T13[])
                n152 = call "Log One-Second Interval Message (if necessary).vi"("error in (no error)"=w353, "Errors in current one-second interval"=w351) -> ("error out"=w352:errorcluster)  [unwired: 9 in]
                n153 = Bundle By Name(cluster=w349, "Errors in current one-second interval"=w348) -> (w350:T10)
              }
            }
            n154 = call "Handle Internal Error.vi"("error in (no error)"=w121) -> ("error out"=w120:errorcluster)  [unwired: 10 in]
            "MHL iteration" <- w123
          }
          n155 = while "\"Log to File\" Loop" {
            shift-right: [w51] -> w25
            shift-left: w24 -> [w56]
            stop <- w53 stop-if-true
            # "A dedicated logging loop was created in order to remove the burden of a lengthy, time-consuming, sequential (blocking) operation from the MHL loop. So that the MHL has more time to deal with other things. A dedicated logging loop is judged to improve the overall performance of the Error Handler (the number of errors that can be logged to file per second)."
            n156 = call "Dequeue.vi"("error in (no error)"=w56) -> ("error out"=w55:errorcluster, "Data"=w50:variant, "Command"=w54:T3)  [unwired: 8 in]
            n157 = case shown="\"Log Error\"" w54 {
              tunnel: w55 -> [w57 w60 w66]
              tunnel: [_ TRUE _] -> w53
              tunnel: [w57 w58 w67] -> w52
              tunnel: w50 -> [_ _ w64]
              frame "Init Loop" {
              }
              frame "Close Loop" {
                n158 = call "Destroy.vi"("error in (no error)"=w60) -> ("error out"=w59:errorcluster)  [unwired: 8 in, 2 out]
                n159 = Merge Errors(w60, w59) -> (w58:errorcluster)
              }
              frame "Log Error" {
                n160 = Variant To Data(error in=w66, type=T5 {"Error Type"=enum."New", "Error Number"=0, "Timestamp"=timestamp(0 s since 1904-01-01), "Error code"=0, "Error message"=""} ("Error to be logged"), Variant=w64) -> (data=w62:T5, error out=w65:errorcluster)
                n161 = call "Write Error.vi"("error in (no error)"=w65, "Error to be logged"=w62) -> ("error out"=w67:errorcluster)  [unwired: 9 in]
              }
            }
            n162 = call "Handle Internal Error.vi"("error in (no error)"=w52) -> ("error out"=w51:errorcluster)  [unwired: 10 in]
          }
          n163 = while "\"New Error Dialogue\" Loop" {
            shift-right: [w36] -> w23
            shift-left: w24 -> [w38]
            stop <- w32 stop-if-true
            n164 = call "Dequeue.vi"("error in (no error)"=w38) -> ("error out"=w35:errorcluster, "Data"=w33:variant, "Command"=w34:T2)  [unwired: 8 in]
            n165 = case shown="\"Pop-up New Error Dialogue\"" w34 {
              tunnel: w35 -> [w39 w40 w49]
              tunnel: [w39 w43 w48] -> w37
              tunnel: w33 -> [_ _ w46]
              tunnel: [_ TRUE _] -> w32
              frame "Init Loop" {
              }
              frame "Close Loop" {
                n166 = call "Destroy.vi"("error in (no error)"=w40) -> ("error out"=w41:errorcluster)  [unwired: 8 in, 2 out]
                n167 = Merge Errors(w40, w41) -> (w43:errorcluster)
              }
              frame "Pop-up New Error Dialogue" {
                w45 = T14 {"Error Code"=0, "Error Message"=""}  # New Error
                n168 = Variant To Data(error in=w49, type=w45, Variant=w46) -> (data=w44:T14, error out=w47:errorcluster)
                n169 = call "Main.vi"("Error In"=w47, "New Error (To Be Displayed To User)"=w44) -> ("Error Out"=w48:errorcluster)  [unwired: 9 in]
              }
            }
            n170 = call "Handle Internal Error.vi"("error in (no error)"=w37) -> ("error out"=w36:errorcluster)  [unwired: 10 in]
          }
          n171 = while "Metronome Loop" {
            shift-right: [w358] -> _
            shift-left: w28 -> [w357]
            shift-right: [w355] -> w27
            shift-left: w24 -> [w356]
            stop <- w365 stop-if-true
            w361 = 1.0  # Metronome period (seconds)
            # "Determines the frequency at which the loop checks whether the interval has elapsed or not."
            n172 = Get Date/Time In Seconds() -> (seconds since 1Jan1904=w359:timestamp)
            n173 = To Double Precision Float(number=w359) -> (double precision float=w364:dbl)
            n174 = To Double Precision Float(number=w357) -> (double precision float=w363:dbl)
            n175 = Subtract(x=w364, y=w363) -> (x-y=w362:dbl)
            n176 = Greater Or Equal?(x=w362, y=w361) -> (x >= y?=w360:bool)
            n177 = case shown="True" w360 {
              tunnel: w359 -> [_ w373]
              tunnel: [w369 w373] -> w358
              tunnel: w357 -> [w369 _]
              tunnel: w356 -> [w368 w372]
              tunnel: [w368 w371] -> w354
              frame False {
                # "We are still in the existing one-second interval"
              }
              frame True {
                # "The one-second interval active until now has just expired."
                # "Update the one-second interval start time"
                # "The start of a new one-second interval"
                n178 = call "Enqueue High Priority.vi"("error in (no error)"=w372, "Command"=Command_(enum)."One-Second Interval Expired") -> ("error out"=w371:errorcluster)  [unwired: 9 in]
              }
            }
            n179 = flat-sequence {
              tunnel: [w366] -> w355
              tunnel: w354 -> [w366]
              frame #0 {
                n180 = Wait (ms)(milliseconds to wait=u32 50) -> ()  [unwired: 1 out]
              }
            }
            n181 = local read "Close module?"() -> (w365:bool)
          }
          n182 = call <vilib>:"Clear Errors.vi"("error in (no error)"=w27) -> ("error out"=w22:errorcluster)  [unwired: 5 in, 1 out]
          n183 = Merge Errors(w29, w31, w25, w23, w22) -> (w30:errorcluster)
        }
        frame Error {
          w374 = T15 1 items=["no dialog", "OK message", "continue or stop message", "OK message + warnings", "continue/stop + warnings"] ("type of dialog (OK msg:1)")
          # "Error during pre-loop initialisation. Exit VI."
          n184 = call <vilib>:"Simple Error Handler.vi"("type of dialog (OK msg:1)"=w374, "error in (no error)"=w376) -> ("error out"=w375:errorcluster)  [unwired: 3 in, 4 out]
        }
      }
    }
    frame Error {
    }
  }
  "Error Out" <- w2
